vi "EditOptions.vi"(8 "error in":errorcluster, 11 "node in":refnum<class "RunTimeObjectsSection.lvclass">) -> (0 "error out":errorcluster, 1 "edit options":T1, 2 "subnodes class":T2, 3 "node out":refnum<class "RunTimeObjectsSection.lvclass">)   [LabVIEW 2015, in "RunTimeObjectsSection.lvclass"]
doc: "Contains the options for the Menu that will be displayed when doing right click on an item.\nThe sub nodes class configures which nodes can be added to this nodes\nAnd the edit options determine which options are available for the node.\nThis configuration is stored in this VI in case some dynamic configuration is required for the menu options or sub nodes."
uses:
  RunTimeObjectsSection.lvclass
  <vilib>/NI/Configuration Framework/Node/SubNodeCluster.ctl
  <vilib>/NI/Configuration Framework/Node/NodeMenuOptions.ctl
  RunTimeObjectsSection.lvclass/RunTimeObjectsSection.ctl
  <vilib>/NI/Configuration Framework/Node/NISE_CEF_Node.lvclass/NISE_CEF_Node.ctl
  ActionVI/ActionVI.lvclass
  ActionVI/ActionVI.lvclass/ActionVI.ctl
  ActionVI/Read ActionVIType.vi
  <vilib>/NI/Configuration Framework/Node/ReadChildren.vi
  <vilib>/NI/Configuration Framework/Node/NISE_CEF_Node.lvclass
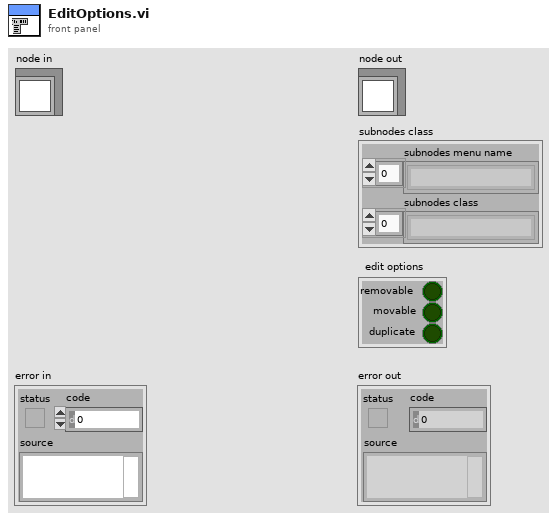
[diagram p1: front panel]
types:
  T1 = typedef "NISE_CEF_Node.lvclass/NodeMenuOptions.ctl" = cluster{"removable":bool, "movable":bool, "duplicate":bool}
  T2 = typedef "NISE_CEF_Node.lvclass/SubNodeCluster.ctl" = cluster{"subnodes menu name":string[], "subnodes class":string[]}
  T3 = typedef "Configuration Tool.lvlib/RunTimeObjectTypes.ctl" = enum16{"ActionVIs", "ButtonList", "RunTimeMenu"}
  T4 = typedef "NISE_CEF_Node.lvclass/NodeRef.ctl" = refnum<data-value>
  T5 = typedef "Configuration Tool.lvlib/ActionVITypes.ctl" = enum16{"OnDelete", "OnLoad", "OnPaste", "OnTargetTypeChange", "OnDeleteRequest", "OnCompile", "OnSystemShutdown", "OnSave", "OnDownload"}
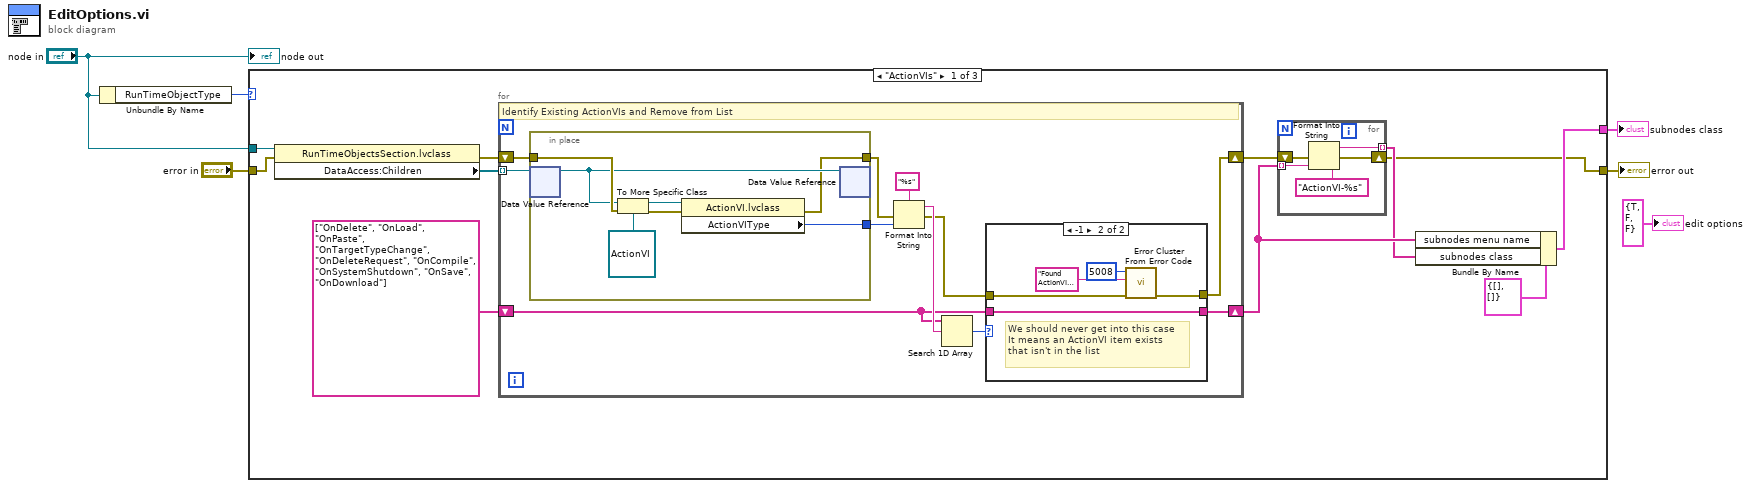
[diagram p0: block diagram]
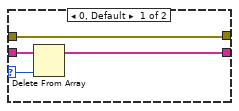
[diagram p2: hidden frame]
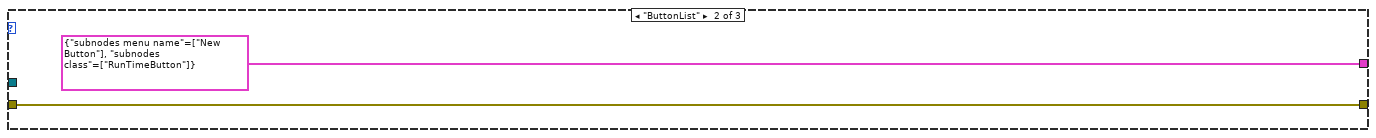
[diagram p3: hidden frame]
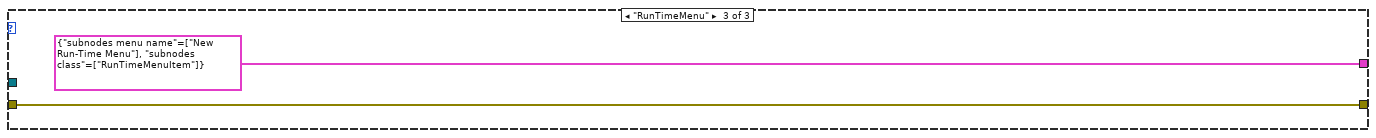
[diagram p4: hidden frame]
diagram:
  n1 = Unbundle By Name("node in") -> ("RunTimeObjectType"=w5:T3)
  n2 = case shown="\"ActionVIs\"" w5 {
    tunnel: [w8 T2 {"subnodes menu name"=["New Button"], "subnodes class"=["RunTimeButton"]} ("subnodes class") T2 {"subnodes menu name"=["New Run-Time Menu"], "subnodes class"=["RunTimeMenuItem"]} ("subnodes class")] -> w4
    tunnel: "node in" -> [w17 _ _]
    tunnel: "error in" -> [w16 w50 w52]
    tunnel: [w7 w50 w52] -> w1
    frame "ActionVIs" {
      n3 = property class="RunTimeObjectsSection.lvclass"(reference=w17, error in=w16) -> (error out=w14:errorcluster, "DataAccess:Children"=w15:T4[])  [unwired: 1 out]
      n4 = for {
        tunnel: w15 -> [w28] mode=indexing
        shift-right: [w18] -> w13
        shift-left: w14 -> [w27]
        shift-right: [w21] -> w10
        shift-left: string[] ["OnDelete", "OnLoad", "OnPaste", "OnTargetTypeChange", "OnDeleteRequest", "OnCompile", "OnSystemShutdown", "OnSave", "OnDownload"] ("Array") -> [w22]
        # "Identify Existing ActionVIs and Remove from List"
        n5 = in-place {
          in-place-border: w27 -> [w44]
          in-place-border: [w39] -> w25
          in-place-border: [w38] -> w26
          n6 = in-place-dvr #1(w28) -> (w40:refnum<class "NISE_CEF_Node.lvclass">)  [unwired: 1 out]
          n7 = To More Specific Class(target class=refnum<class "ActionVI.lvclass"> refnum ("ActionVI.lvclass"), reference=w40, error in=w44) -> (specific class reference=w42:refnum<class "ActionVI.lvclass">, error out=w41:errorcluster)
          n8 = property class="ActionVI.lvclass"(reference=w42, error in=w41) -> (error out=w39:errorcluster, "ActionVIType"=w38:T5)  [unwired: 1 out]
          n9 = in-place-dvr #1(w40) -> ()  [unwired: 2 out]
        }
        n10 = Format Into String(format string="%s", error in=w25, w26) -> (resulting string=w23:string, error out=w19:errorcluster)  [unwired: 1 in]
        n11 = Search 1D Array(1D array=w22, element=w23) -> (index of element=w20:i32)  [unwired: 1 in]
        n12 = case shown="-1" w20 {
          selector: w20 -> [w30 _]
          tunnel: w22 -> [w32 w37]
          tunnel: [w31 w37] -> w21
          tunnel: w19 -> [w29 w36]
          tunnel: [w29 w33] -> w18
          frame 0, Default {
            n13 = Delete From Array(array=w32, index=w30) -> (array with subset deleted=w31:string[])  [unwired: 1 in, 1 out]
          }
          frame -1 {
            # "We should never get into this case\nIt means an ActionVI item exists\nthat isn't in the list"
            n14 = call <vilib>:"Error Cluster From Error Code.vi"("error in (no error)"=w36, "error message (\"\")"="Found ActionVI object that we weren't expecting" ("error message (\"\")"), "error code (0)"=5008) -> ("error out"=w33:errorcluster)  [unwired: 6 in]
          }
        }
      }
      n15 = for {
        tunnel: w10 -> [w49] mode=indexing
        shift-right: [w46] -> w7
        shift-left: w13 -> [w47]
        tunnel: [w45] -> w9 mode=indexing
        n16 = Format Into String(format string="ActionVI-%s", error in=w47, w49) -> (resulting string=w45:string, error out=w46:errorcluster)  [unwired: 1 in]
      }
      n17 = Bundle By Name(cluster=T2 {"subnodes menu name"=[], "subnodes class"=[]} ("subnodes class"), "subnodes menu name"=w10, "subnodes class"=w9) -> (w8:T2)
    }
    frame "ButtonList" {
    }
    frame "RunTimeMenu" {
    }
  }
  "error out" <- w1
  "subnodes class" <- w4
  "node out" <- "node in"
  "edit options" <- T1 {"removable"=TRUE, "movable"=FALSE, "duplicate"=FALSE} ("edit options")
